vi "INIT.vi"(8 "error in (no error)":errorcluster, 11 "TELEDINE_LECROY in":refnum<class "TELEDINE_LECROY.lvclass">) -> (0 "error out":errorcluster, 3 "TELEDINE_LECROY out":refnum<class "TELEDINE_LECROY.lvclass">)   [LabVIEW 2020, in "TELEDINE_LECROY.lvclass"]
uses:
  TELEDINE_LECROY.lvclass
  C:/dev/TRANCON/Classes/GeneralFunctionality/GeneralFunctionality.lvclass
  GeneralFunctionality/GeneralFunctionality.lvclass/GeneralFunctionality.ctl
  GeneralFunctionality/GeneralFunctionality.lvclass
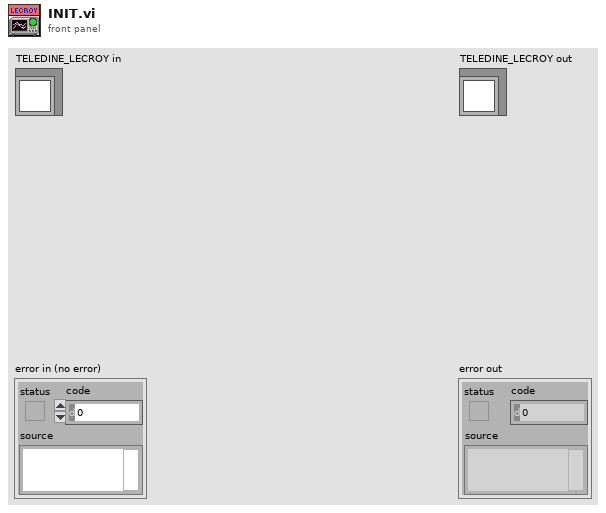
[diagram p1: front panel]
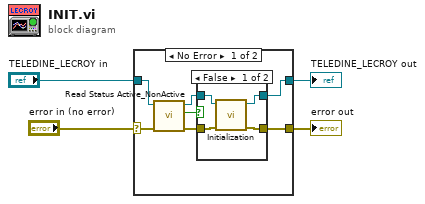
[diagram p0: block diagram]
diagram:
  n1 = case shown="No Error" "error in (no error)" {
    selector: "error in (no error)" -> [w6 w19]
    tunnel: [w11 w18] -> w2
    tunnel: [w10 w19] -> w1
    tunnel: "TELEDINE_LECROY in" -> [w9 w18]
    frame No Error {
      n2 = call "Read Status Active_NonActive.vi"("error in (no error)"=w6, "GeneralFunctionality in"=w9) -> ("error out"=w5:errorcluster, "Status Active/NonActive"=w8:bool, "GeneralFunctionality out"=w7:refnum<class "TELEDINE_LECROY.lvclass">)  [unwired: 7 in]
      n3 = case shown="False" w8 {
        tunnel: [w13 w17] -> w11
        tunnel: [w12 w16] -> w10
        tunnel: w7 -> [w15 w17]
        tunnel: w5 -> [w14 w16]
        frame False {
          n4 = call "Initialization.vi"("error in (no error)"=w14, "TELEDINE_LECROY in"=w15) -> ("error out"=w12:errorcluster, "TELEDINE_LECROY out"=w13:refnum<class "TELEDINE_LECROY.lvclass">)  [unwired: 8 in]
        }
        frame True {
        }
      }
    }
    frame Error {
    }
  }
  "error out" <- w1
  "TELEDINE_LECROY out" <- w2
